vi "Currents (SubVI).vi"() -> (6 "Shooter Current":dbl(graph), 7 "String 5":string, 8 "lf drive I":string, 9 "String 4":string, 10 "lr drive I":string, 11 "String 3":string, 12 "String":string, 13 "String 9":string, 14 "String 2":string, 15 "String 7":string, 16 "String 10":string, 17 "String 6":string, 18 "String 8":string)   [LabVIEW 2015]
uses:
  <vilib>/Rock Robotics/Network Tables/NT Read Number.vi
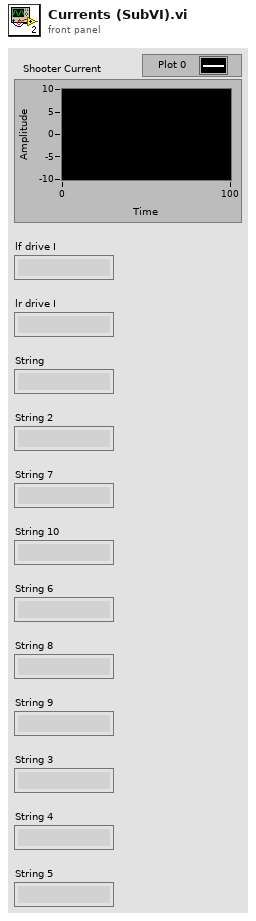
[diagram p1: front panel]
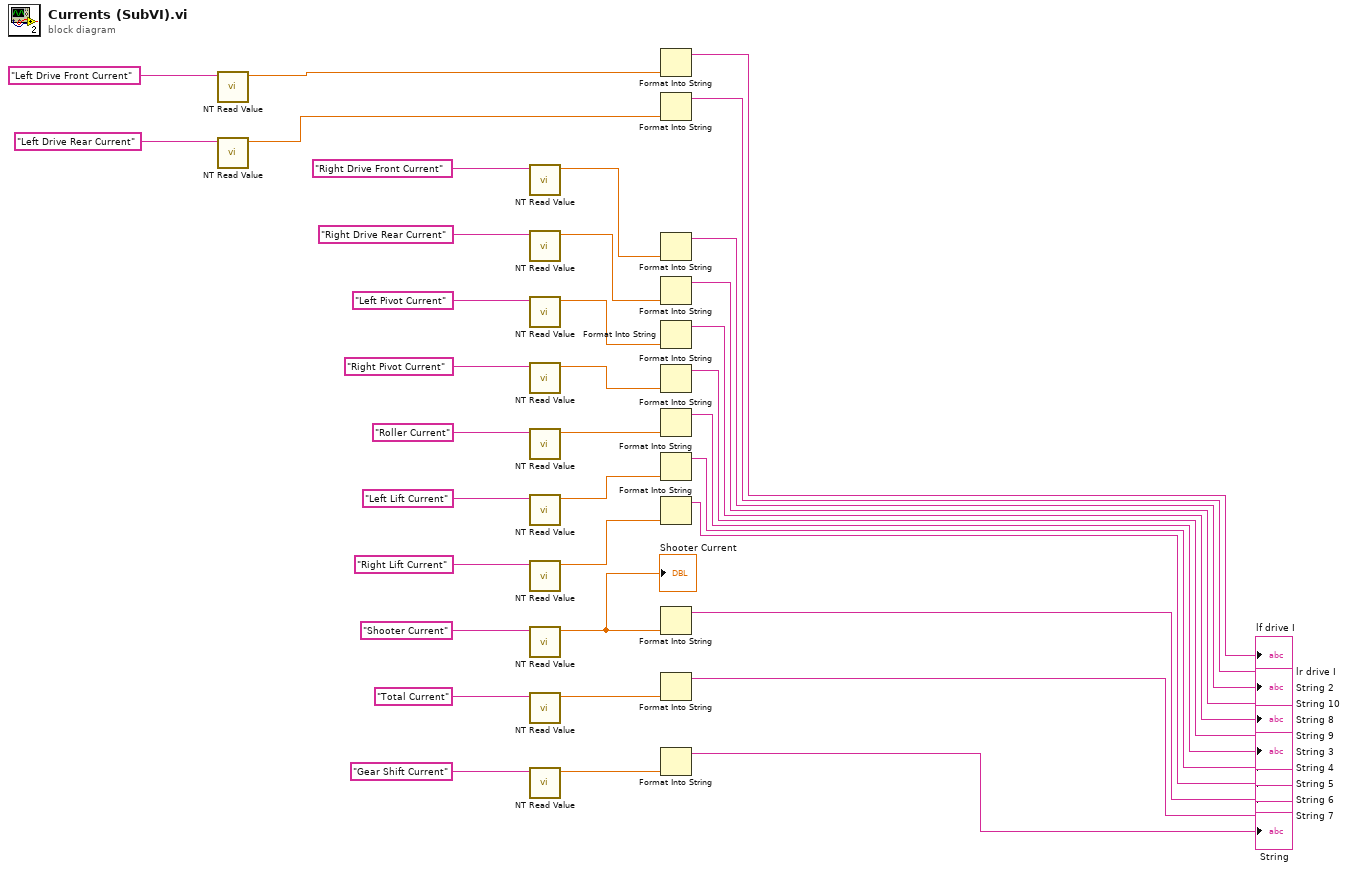
[diagram p0: block diagram]
diagram:
  n1 = call-poly <vilib>:"NT Read Value.vi"("Name"="Left Drive Front Current") -> ("Numeric"=w7:dbl)  [unwired: 9 in, 1 out]
  n2 = call-poly <vilib>:"NT Read Value.vi"("Name"="Left Drive Rear Current") -> ("Numeric"=w5:dbl)  [unwired: 9 in, 1 out]
  n3 = call-poly <vilib>:"NT Read Value.vi"("Name"="Right Drive Front Current") -> ("Numeric"=w23:dbl)  [unwired: 9 in, 1 out]
  n4 = call-poly <vilib>:"NT Read Value.vi"("Name"="Right Drive Rear Current") -> ("Numeric"=w21:dbl)  [unwired: 9 in, 1 out]
  n5 = call-poly <vilib>:"NT Read Value.vi"("Name"="Left Pivot Current") -> ("Numeric"=w19:dbl)  [unwired: 9 in, 1 out]
  n6 = call-poly <vilib>:"NT Read Value.vi"("Name"="Right Pivot Current") -> ("Numeric"=w17:dbl)  [unwired: 9 in, 1 out]
  n7 = call-poly <vilib>:"NT Read Value.vi"("Name"="Roller Current") -> ("Numeric"=w15:dbl)  [unwired: 9 in, 1 out]
  n8 = call-poly <vilib>:"NT Read Value.vi"("Name"="Left Lift Current") -> ("Numeric"=w13:dbl)  [unwired: 9 in, 1 out]
  n9 = call-poly <vilib>:"NT Read Value.vi"("Name"="Right Lift Current") -> ("Numeric"=w11:dbl)  [unwired: 9 in, 1 out]
  n10 = call-poly <vilib>:"NT Read Value.vi"("Name"="Shooter Current") -> ("Numeric"=w33:dbl)  [unwired: 9 in, 1 out]
  "Shooter Current" <- w33
  n11 = call-poly <vilib>:"NT Read Value.vi"("Name"="Total Current") -> ("Numeric"=w8:dbl)  [unwired: 9 in, 1 out]
  n12 = call-poly <vilib>:"NT Read Value.vi"("Name"="Gear Shift Current") -> ("Numeric"=w34:dbl)  [unwired: 9 in, 1 out]
  n13 = Format Into String(w7) -> (resulting string=→"lf drive I":string)  [unwired: 3 in, 1 out]
  n14 = Format Into String(w5) -> (resulting string=→"lr drive I":string)  [unwired: 3 in, 1 out]
  n15 = Format Into String(w23) -> (resulting string=→"String 2":string)  [unwired: 3 in, 1 out]
  n16 = Format Into String(w21) -> (resulting string=→"String 10":string)  [unwired: 3 in, 1 out]
  n17 = Format Into String(w19) -> (resulting string=→"String 8":string)  [unwired: 3 in, 1 out]
  n18 = Format Into String(w17) -> (resulting string=→"String 9":string)  [unwired: 3 in, 1 out]
  n19 = Format Into String(w15) -> (resulting string=→"String 3":string)  [unwired: 3 in, 1 out]
  n20 = Format Into String(w13) -> (resulting string=→"String 4":string)  [unwired: 3 in, 1 out]
  n21 = Format Into String(w11) -> (resulting string=→"String 5":string)  [unwired: 3 in, 1 out]
  n22 = Format Into String(w33) -> (resulting string=→"String 6":string)  [unwired: 3 in, 1 out]
  n23 = Format Into String(w8) -> (resulting string=→"String 7":string)  [unwired: 3 in, 1 out]
  n24 = Format Into String(w34) -> (resulting string=→"String":string)  [unwired: 3 in, 1 out]
